vi "niRFUtil WFM Correlate (real array).vi"(1 "Reference Array In":T1 min=0 max=127 format="%.2f", 2 "Array In":T1 min=0 max=127 format="%.2f") -> (0 "Array Out":T1 min=0 max=127 format="%.2f")   [LabVIEW 2015, in "niRFUtil.lvlib"]
doc: "(c) Copyright 2006, National Instruments, Inc. This VI may not be duplicated, sold, or distributed without written consent from National Instruments."
uses:
  niRFUtil.lvlib
  Includes/niRFUtil INC Real Array.ctl
  <vilib>/Analysis/2dsp.llb/1D Cross Correlation (DBL).vi
  <vilib>/Analysis/NI_AALPro.lvlib
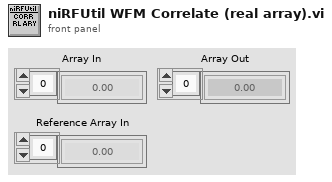
[diagram p1: front panel]
types:
  T1 = typedef "niRFUtil.lvlib/niRFUtil INC Real Array.ctl" = sgl[]
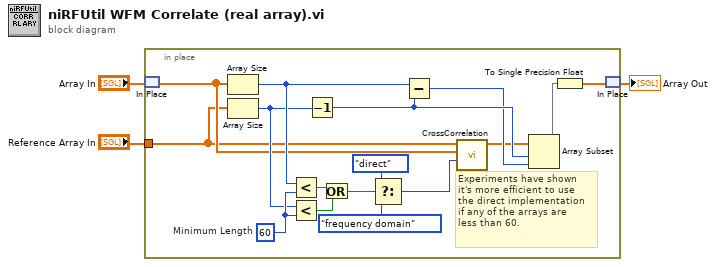
[diagram p0: block diagram]
diagram:
  n1 = in-place {
    in-place-border: "Reference Array In" -> [w4]
    w19 = 60  # Minimum Length
    # "Experiments have shown\nit's more efficient to use\nthe direct implementation\nif any of the arrays are\nless than 60."
    n2 = in-place-match #1("Array In") -> (w6:T1)
    n3 = Array Size(array=w6) -> (size(s)=w10:i32)
    n4 = Array Size(array=w4) -> (size(s)=w9:i32)
    n5 = Less?(x=w10, y=w19) -> (x < y?=w18:bool)
    n6 = Less?(x=w9, y=w19) -> (x < y?=w17:bool)
    n7 = Decrement(x=w9) -> (x-1=w12:i32)
    n8 = Or(x=w18, y=w17) -> (x .or. y?=w16:bool)
    n9 = Select(t=enum32{"direct", "frequency domain"}."direct" ("algorithm"), s=w16, f=enum32{"direct", "frequency domain"}."frequency domain" ("algorithm")) -> (s? t:f=w7:enum32{"direct", "frequency domain"})
    n10 = Subtract(x=w10, y=w12) -> (x-y=w11:i32)
    n11 = call-poly <vilib>:"CrossCorrelation.vi"("algorithm"=w7, "Y"=w6, "X"=w4) -> ("Rxy"=w8:dbl[])  [unwired: 7 in, 1 out]
    n12 = Array Subset(array=w8, index=w12, length=w11) -> (w13:dbl[])
    n13 = To Single Precision Float(number=w13) -> (single precision float=w5:sgl[])
    n14 = in-place-match #1(w5) -> (→"Array Out":T1)
  }
